vi "Add New Group.vi"(0 "Node Ptr":T1 format="%.0x") -> ()   [LabVIEW 2024, in "Embedded TDMS Logger System Explorer.lvlib"]
doc: "Adds a new group section to the System Definition of the Custom Device appended to the end."
uses:
  Embedded TDMS Logger System Explorer.lvlib
  <vilib>/NI VeriStand/Custom Device API/Custom Device Item Ref.ctl
  Shared/Constants.vi
  <vilib>/NI VeriStand/Custom Device API/Set Item Property (Boolean).vi
  <vilib>/NI VeriStand/Custom Device API/Custom Device API.lvlib
  Shared/Embedded TDMS Logger Shared.lvlib
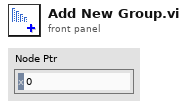
[diagram p1: front panel]
types:
  T1 = typedef "Custom Device API.lvlib/Custom Device Item Ref.ctl" = u64
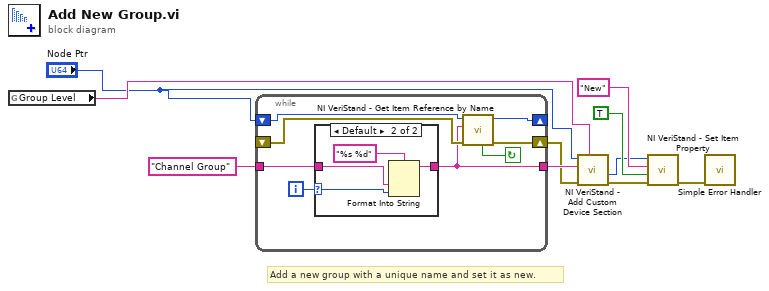
[diagram p0: block diagram]
diagram:
  # "Add a new group with a unique name and set it as new."
  n1 = global read "Constants.vi" "Group Level"() -> (w10:string)
  n2 = while {
    shift-right: [w12] -> w7
    shift-left: _ -> [w16]
    shift-right: [w14] -> _
    shift-left: "Node Ptr" -> [w15]
    tunnel: "Channel Group" ("group name") -> [w17]
    tunnel: [w11] -> w8
    i -> [w18]
    stop <- w13 continue-if-true
    n3 = case shown="Default" w18 {
      selector: w18 -> [_ w21]
      tunnel: w17 -> [w19 w22]
      tunnel: [w19 w20] -> w11
      frame 0 {
      }
      frame Default {
        n4 = Format Into String(format string="%s %d", w22, w21) -> (resulting string=w20:string)  [unwired: 2 in, 1 out]
      }
    }
    n5 = call <vilib>:"NI VeriStand - Get Item Reference by Name.vi"("error in (no error)"=w16, "Item Name"=w11, "Parent Ref in"=w15) -> ("error out"=w12:errorcluster, "Parent Ref out"=w14:T1, "Found"=w13:bool)  [unwired: 6 out]
  }
  n6 = call <vilib>:"NI VeriStand - Add Custom Device Section.vi"("GUID (Default Section)"=w10, "error in (no error)"=w7, "Section Name"=w8, "Parent Ref in"="Node Ptr") -> ("error out"=w3:errorcluster, "Section Ptr"=w2:T1)  [unwired: 3 in, 3 out]
  n7 = call-poly <vilib>:"NI VeriStand - Set Item Property.vi"("error in (no error)"=w3, "Value"=TRUE, "Property Name"="New", "Item Ref in"=w2) -> ("error out"=w4:errorcluster)  [unwired: 5 in, 2 out]
  n8 = call <vilib>:"Simple Error Handler.vi"("error in (no error)"=w4) -> ()  [unwired: 4 in, 5 out]
